vi "PianoPassiveBuzzer.vi"() -> ()   [LabVIEW 2024]
uses:
  Driver/CTIPicoVISA.lvlib
panel:
  in  "GroveConnector":enum16{"A0", "A1", "A2"}(ring)
  out "error out":errorcluster
  out "Identity":T1
  in  "Duty Cycle":dbl(slide)=0.09183673469387754 scale=0.0..1.0
  in  "D5#":bool
  in  "E5":bool
  in  "C5#":bool
  in  "D5":bool
  in  "A4#":bool
  in  "G4#":bool
  in  "F4#":bool
  in  "D4#":bool
  in  "C4#":bool
  in  "VISA resource":refnum<visa-resource-name>="ASRL5::INSTR"
  in  "stop":bool
  in  "C5":bool
  in  "B4":bool
  in  "A4":bool
  in  "G4":bool
  in  "F4":bool
  in  "E4":bool
  in  "D4":bool
  in  "C4":bool
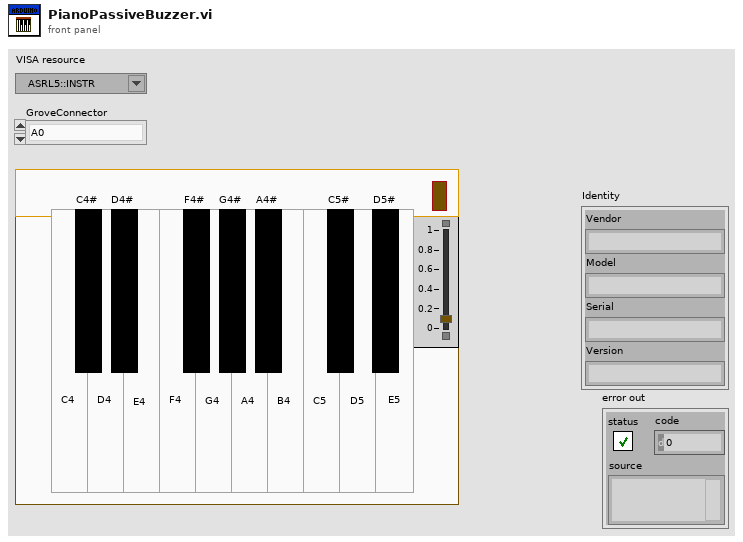
[diagram p1: front panel]
types:
  T1 = cluster{"Vendor":string, "Model":string, "Serial":string, "Version":string}
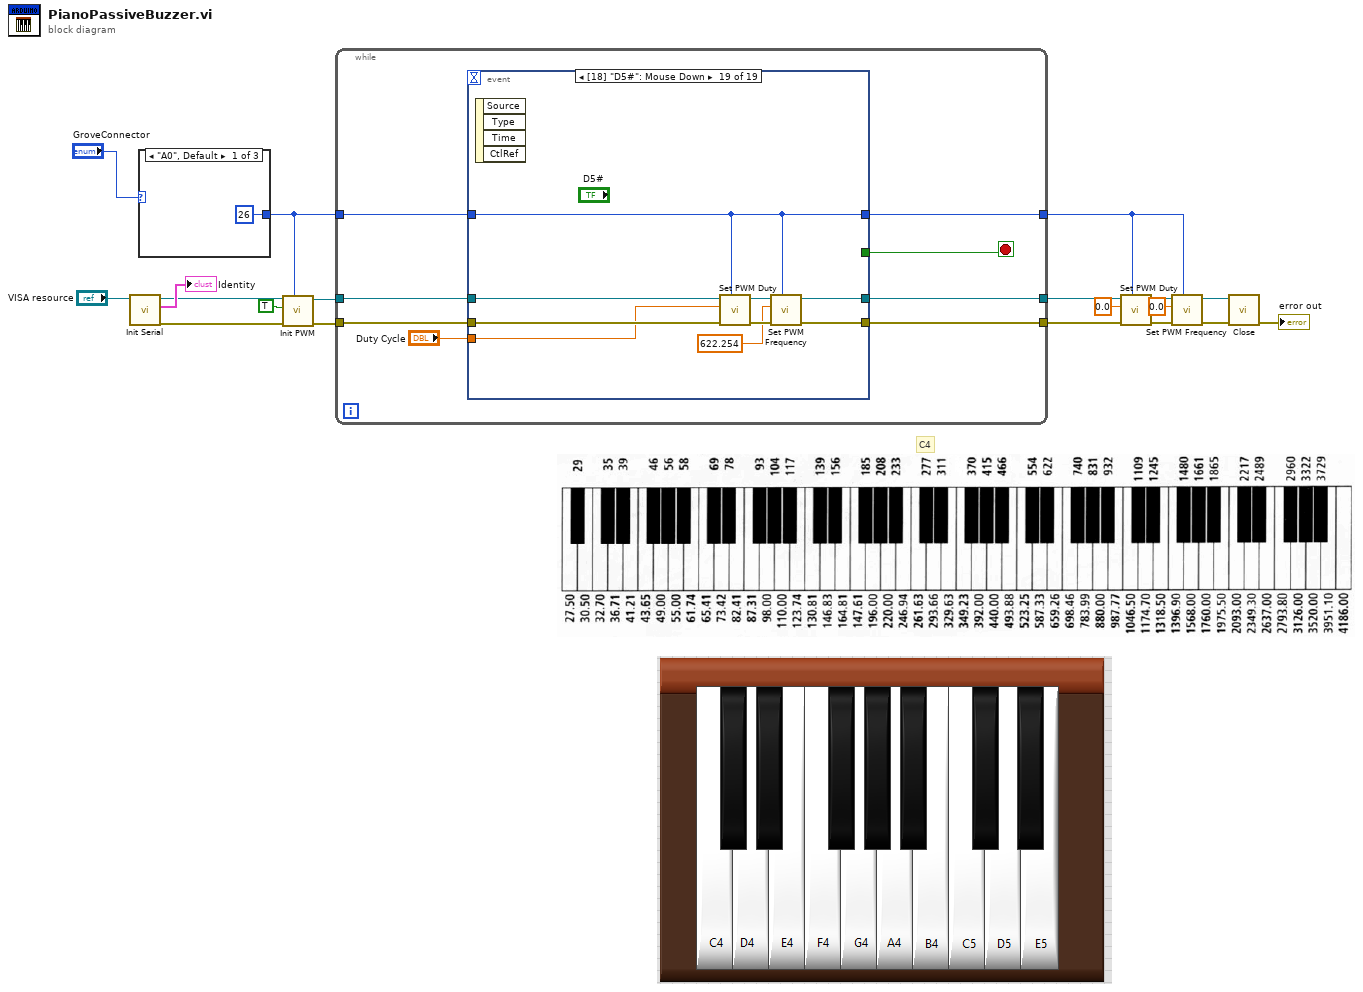
[diagram p0: block diagram]
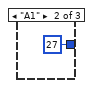
[diagram p2: hidden frame]
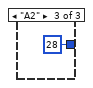
[diagram p3: hidden frame]
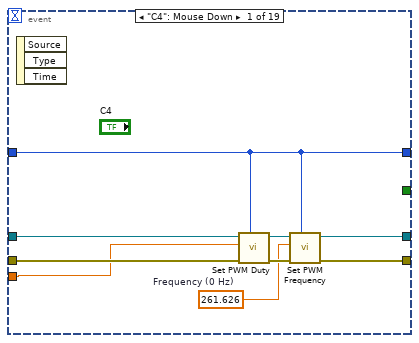
[diagram p4: hidden frame]
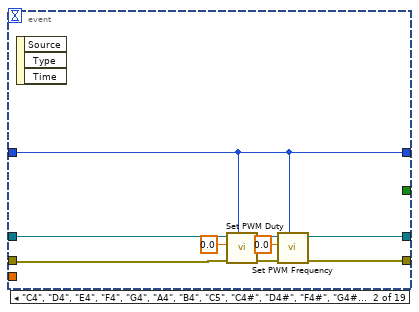
[diagram p5: hidden frame]
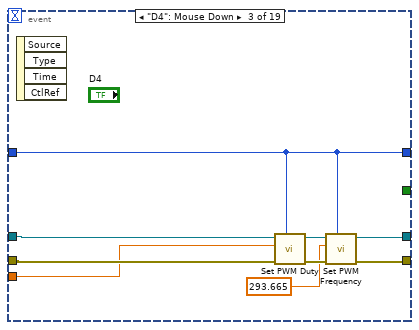
[diagram p6: hidden frame]
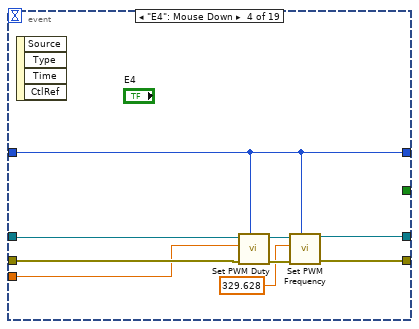
[diagram p7: hidden frame]
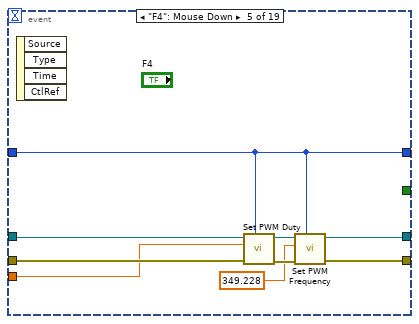
[diagram p8: hidden frame]
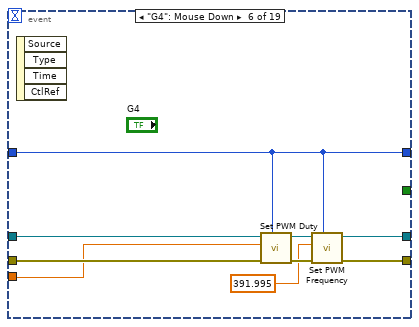
[diagram p9: hidden frame]
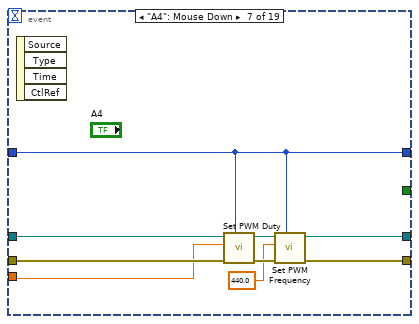
[diagram p10: hidden frame]
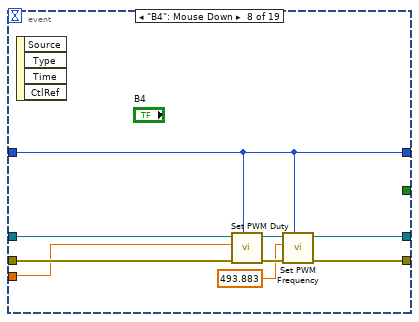
[diagram p11: hidden frame]
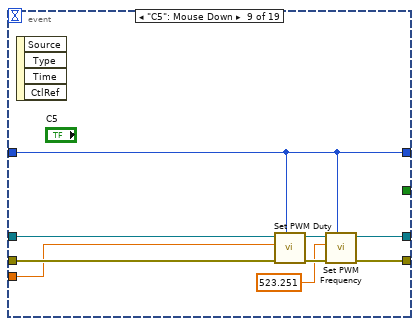
[diagram p12: hidden frame]
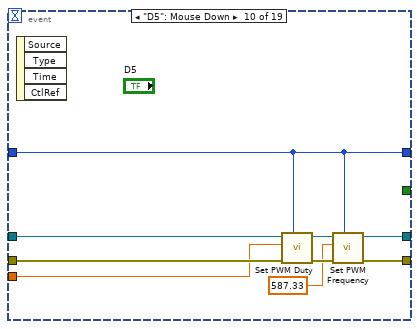
[diagram p13: hidden frame]
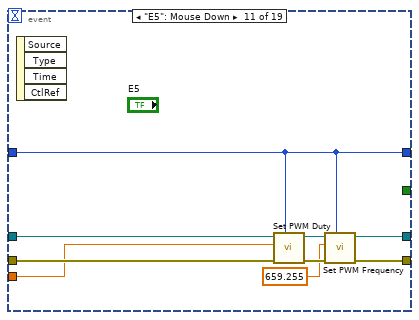
[diagram p14: hidden frame]
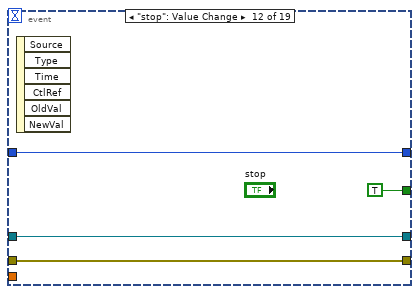
[diagram p15: hidden frame]
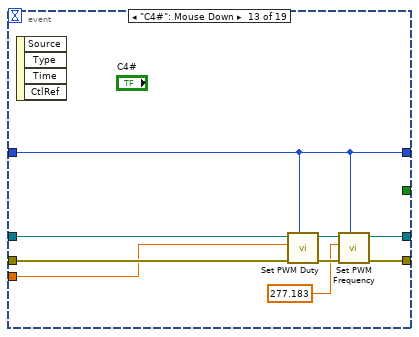
[diagram p16: hidden frame]
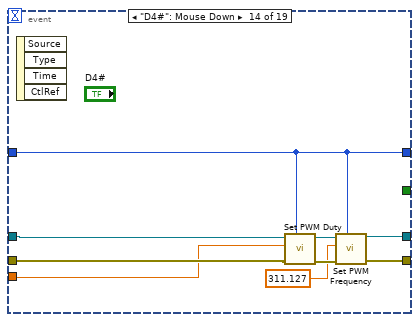
[diagram p17: hidden frame]
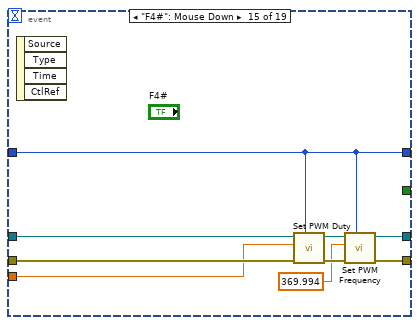
[diagram p18: hidden frame]
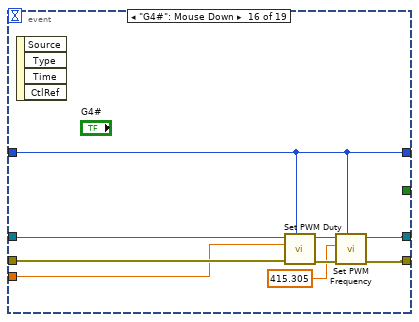
[diagram p19: hidden frame]
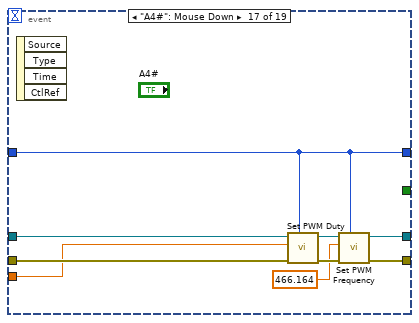
[diagram p20: hidden frame]
diagram:
  # "C4"
  n1 = call "Init Serial.vi"("VISA resource name in"="VISA resource") -> ("error out"=w12:errorcluster, "Identity"=→"Identity":T1, "VISA resource name Out"=w11:refnum<visa-resource-name>)  [unwired: 8 in]
  n2 = case shown="\"A0\", Default" "GroveConnector" {
    tunnel: [26 ("GPIO") 27 ("GPIO") 28 ("GPIO")] -> w2
    frame "A0", Default {
    }
    frame "A1" {
    }
    frame "A2" {
    }
  }
  n3 = call "Init PWM.vi"("GPIO"=w2, "error in (no error)"=w12, "Enable (F)"=TRUE, "VISA resource name in"=w11) -> ("error out"=w13:errorcluster, "VISA resource name"=w14:refnum<visa-resource-name>)  [unwired: 6 in]
  n4 = while {
    tunnel: w14 -> [w29]
    tunnel: w13 -> [w28]
    tunnel: [w25] -> w5
    tunnel: [w26] -> w6
    tunnel: w2 -> [w24]
    tunnel: [w23] -> w1
    stop <- w27 stop-if-true
    n5 = event shown="[18] \"D5#\": Mouse Down" {
      selector: _ -> [_ _ _ _ _ _ _ _ _ _ _ _ _ _ _ _ _ _ _]
      dyn-events: _ -> [_ _ _ _ _ _ _ _ _ _ _ _ _ _ _ _ _ _ _]
      timeout: _ -> [_ _ _ _ _ _ _ _ _ _ _ _ _ _ _ _ _ _ _]
      tunnel: "Duty Cycle" -> [w31 _ w49 w58 w68 w77 w85 w94 w103 w112 w122 _ w136 w144 w152 w162 w170 w179 w188]
      tunnel: w29 -> [w34 w44 w50 w62 w70 w79 w88 w98 w106 w115 w124 w132 w135 w146 w156 w164 w174 w183 w192]
      tunnel: w28 -> [w35 w43 w52 w61 w69 w78 w89 w97 w105 w114 w123 w131 w137 w145 w155 w163 w173 w182 w191]
      tunnel: [w36 w45 w54 w63 w72 w81 w90 w99 w108 w116 w126 w131 w139 w148 w157 w166 w175 w184 w193] -> w25
      tunnel: [w37 w46 w55 w64 w73 w82 w91 w100 w109 w118 w127 w132 w140 w149 w158 w167 w176 w185 w194] -> w26
      tunnel: [_ _ _ _ _ _ _ _ _ _ _ TRUE _ _ _ _ _ _ _] -> w27
      tunnel: w24 -> [w33 w40 w53 w60 w71 w80 w87 w96 w107 w117 w125 w130 w134 w147 w154 w165 w172 w181 w190]
      tunnel: [w33 w40 w53 w60 w71 w80 w87 w96 w107 w117 w125 w130 w134 w147 w154 w165 w172 w181 w190] -> w23
      event "C4": Mouse Down {
        w32 = 261.626  # Frequency (0 Hz)
        n6 = event-data() -> ()  [unwired: 1 in, 3 out]
        n7 = call "Set PWM Duty.vi"("GPIO"=w33, "error in (no error)"=w35, "Duty % (0-1)"=w31, "VISA resource name in"=w34) -> ("error out"=w39:errorcluster, "VISA resource name"=w38:refnum<visa-resource-name>)  [unwired: 6 in]
        n8 = call "Set PWM Frequency.vi"("GPIO"=w33, "error in (no error)"=w39, "Freq Hz"=w32, "VISA resource name in"=w38) -> ("error out"=w36:errorcluster, "VISA resource name"=w37:refnum<visa-resource-name>)  [unwired: 6 in]
      }
      event "C4", "D4", "E4", "F4", "G4", "A4", "B4", "C5", "C4#", "D4#", "F4#", "G4#", "A4#", "C5#", "D5", "D5#", "E5": Mouse Up {
        n9 = event-data() -> ()  [unwired: 1 in, 3 out]
        n10 = call "Set PWM Duty.vi"("GPIO"=w40, "error in (no error)"=w43, "Duty % (0-1)"=sgl 0.0, "VISA resource name in"=w44) -> ("error out"=w48:errorcluster, "VISA resource name"=w47:refnum<visa-resource-name>)  [unwired: 6 in]
        n11 = call "Set PWM Frequency.vi"("GPIO"=w40, "error in (no error)"=w48, "Freq Hz"=sgl 0.0, "VISA resource name in"=w47) -> ("error out"=w45:errorcluster, "VISA resource name"=w46:refnum<visa-resource-name>)  [unwired: 6 in]
      }
      event "D4": Mouse Down {
        n12 = event-data() -> ()  [unwired: 1 in, 4 out]
        n13 = call "Set PWM Duty.vi"("GPIO"=w53, "error in (no error)"=w52, "Duty % (0-1)"=w49, "VISA resource name in"=w50) -> ("error out"=w57:errorcluster, "VISA resource name"=w56:refnum<visa-resource-name>)  [unwired: 6 in]
        n14 = call "Set PWM Frequency.vi"("GPIO"=w53, "error in (no error)"=w57, "Freq Hz"=293.665 ("Frequency (0 Hz)"), "VISA resource name in"=w56) -> ("error out"=w54:errorcluster, "VISA resource name"=w55:refnum<visa-resource-name>)  [unwired: 6 in]
      }
      event "E4": Mouse Down {
        n15 = event-data() -> ()  [unwired: 1 in, 4 out]
        n16 = call "Set PWM Duty.vi"("GPIO"=w60, "error in (no error)"=w61, "Duty % (0-1)"=w58, "VISA resource name in"=w62) -> ("error out"=w66:errorcluster, "VISA resource name"=w65:refnum<visa-resource-name>)  [unwired: 6 in]
        n17 = call "Set PWM Frequency.vi"("GPIO"=w60, "error in (no error)"=w66, "Freq Hz"=329.628 ("Frequency (0 Hz)"), "VISA resource name in"=w65) -> ("error out"=w63:errorcluster, "VISA resource name"=w64:refnum<visa-resource-name>)  [unwired: 6 in]
      }
      event "F4": Mouse Down {
        n18 = event-data() -> ()  [unwired: 1 in, 4 out]
        n19 = call "Set PWM Duty.vi"("GPIO"=w71, "error in (no error)"=w69, "Duty % (0-1)"=w68, "VISA resource name in"=w70) -> ("error out"=w75:errorcluster, "VISA resource name"=w74:refnum<visa-resource-name>)  [unwired: 6 in]
        n20 = call "Set PWM Frequency.vi"("GPIO"=w71, "error in (no error)"=w75, "Freq Hz"=349.228, "VISA resource name in"=w74) -> ("error out"=w72:errorcluster, "VISA resource name"=w73:refnum<visa-resource-name>)  [unwired: 6 in]
      }
      event "G4": Mouse Down {
        n21 = event-data() -> ()  [unwired: 1 in, 4 out]
        n22 = call "Set PWM Duty.vi"("GPIO"=w80, "error in (no error)"=w78, "Duty % (0-1)"=w77, "VISA resource name in"=w79) -> ("error out"=w84:errorcluster, "VISA resource name"=w83:refnum<visa-resource-name>)  [unwired: 6 in]
        n23 = call "Set PWM Frequency.vi"("GPIO"=w80, "error in (no error)"=w84, "Freq Hz"=391.995, "VISA resource name in"=w83) -> ("error out"=w81:errorcluster, "VISA resource name"=w82:refnum<visa-resource-name>)  [unwired: 6 in]
      }
      event "A4": Mouse Down {
        n24 = event-data() -> ()  [unwired: 1 in, 4 out]
        n25 = call "Set PWM Duty.vi"("GPIO"=w87, "error in (no error)"=w89, "Duty % (0-1)"=w85, "VISA resource name in"=w88) -> ("error out"=w93:errorcluster, "VISA resource name"=w92:refnum<visa-resource-name>)  [unwired: 6 in]
        n26 = call "Set PWM Frequency.vi"("GPIO"=w87, "error in (no error)"=w93, "Freq Hz"=440.0, "VISA resource name in"=w92) -> ("error out"=w90:errorcluster, "VISA resource name"=w91:refnum<visa-resource-name>)  [unwired: 6 in]
      }
      event "B4": Mouse Down {
        n27 = event-data() -> ()  [unwired: 1 in, 4 out]
        n28 = call "Set PWM Duty.vi"("GPIO"=w96, "error in (no error)"=w97, "Duty % (0-1)"=w94, "VISA resource name in"=w98) -> ("error out"=w102:errorcluster, "VISA resource name"=w101:refnum<visa-resource-name>)  [unwired: 6 in]
        n29 = call "Set PWM Frequency.vi"("GPIO"=w96, "error in (no error)"=w102, "Freq Hz"=493.883, "VISA resource name in"=w101) -> ("error out"=w99:errorcluster, "VISA resource name"=w100:refnum<visa-resource-name>)  [unwired: 6 in]
      }
      event "C5": Mouse Down {
        n30 = event-data() -> ()  [unwired: 1 in, 4 out]
        n31 = call "Set PWM Duty.vi"("GPIO"=w107, "error in (no error)"=w105, "Duty % (0-1)"=w103, "VISA resource name in"=w106) -> ("error out"=w111:errorcluster, "VISA resource name"=w110:refnum<visa-resource-name>)  [unwired: 6 in]
        n32 = call "Set PWM Frequency.vi"("GPIO"=w107, "error in (no error)"=w111, "Freq Hz"=523.251, "VISA resource name in"=w110) -> ("error out"=w108:errorcluster, "VISA resource name"=w109:refnum<visa-resource-name>)  [unwired: 6 in]
      }
      event "D5": Mouse Down {
        n33 = event-data() -> ()  [unwired: 1 in, 4 out]
        n34 = call "Set PWM Duty.vi"("GPIO"=w117, "error in (no error)"=w114, "Duty % (0-1)"=w112, "VISA resource name in"=w115) -> ("error out"=w120:errorcluster, "VISA resource name"=w119:refnum<visa-resource-name>)  [unwired: 6 in]
        n35 = call "Set PWM Frequency.vi"("GPIO"=w117, "error in (no error)"=w120, "Freq Hz"=587.33, "VISA resource name in"=w119) -> ("error out"=w116:errorcluster, "VISA resource name"=w118:refnum<visa-resource-name>)  [unwired: 6 in]
      }
      event "E5": Mouse Down {
        n36 = event-data() -> ()  [unwired: 1 in, 4 out]
        n37 = call "Set PWM Duty.vi"("GPIO"=w125, "error in (no error)"=w123, "Duty % (0-1)"=w122, "VISA resource name in"=w124) -> ("error out"=w129:errorcluster, "VISA resource name"=w128:refnum<visa-resource-name>)  [unwired: 6 in]
        n38 = call "Set PWM Frequency.vi"("GPIO"=w125, "error in (no error)"=w129, "Freq Hz"=659.255, "VISA resource name in"=w128) -> ("error out"=w126:errorcluster, "VISA resource name"=w127:refnum<visa-resource-name>)  [unwired: 6 in]
      }
      event "stop": Value Change {
        n39 = event-data() -> ()  [unwired: 1 in, 6 out]
      }
      event "C4#": Mouse Down {
        n40 = event-data() -> ()  [unwired: 1 in, 4 out]
        n41 = call "Set PWM Duty.vi"("GPIO"=w134, "error in (no error)"=w137, "Duty % (0-1)"=w136, "VISA resource name in"=w135) -> ("error out"=w142:errorcluster, "VISA resource name"=w141:refnum<visa-resource-name>)  [unwired: 6 in]
        n42 = call "Set PWM Frequency.vi"("GPIO"=w134, "error in (no error)"=w142, "Freq Hz"=277.183, "VISA resource name in"=w141) -> ("error out"=w139:errorcluster, "VISA resource name"=w140:refnum<visa-resource-name>)  [unwired: 6 in]
      }
      event "D4#": Mouse Down {
        n43 = event-data() -> ()  [unwired: 1 in, 4 out]
        n44 = call "Set PWM Duty.vi"("GPIO"=w147, "error in (no error)"=w145, "Duty % (0-1)"=w144, "VISA resource name in"=w146) -> ("error out"=w151:errorcluster, "VISA resource name"=w150:refnum<visa-resource-name>)  [unwired: 6 in]
        n45 = call "Set PWM Frequency.vi"("GPIO"=w147, "error in (no error)"=w151, "Freq Hz"=311.127, "VISA resource name in"=w150) -> ("error out"=w148:errorcluster, "VISA resource name"=w149:refnum<visa-resource-name>)  [unwired: 6 in]
      }
      event "F4#": Mouse Down {
        n46 = event-data() -> ()  [unwired: 1 in, 4 out]
        n47 = call "Set PWM Duty.vi"("GPIO"=w154, "error in (no error)"=w155, "Duty % (0-1)"=w152, "VISA resource name in"=w156) -> ("error out"=w160:errorcluster, "VISA resource name"=w159:refnum<visa-resource-name>)  [unwired: 6 in]
        n48 = call "Set PWM Frequency.vi"("GPIO"=w154, "error in (no error)"=w160, "Freq Hz"=369.994, "VISA resource name in"=w159) -> ("error out"=w157:errorcluster, "VISA resource name"=w158:refnum<visa-resource-name>)  [unwired: 6 in]
      }
      event "G4#": Mouse Down {
        n49 = event-data() -> ()  [unwired: 1 in, 4 out]
        n50 = call "Set PWM Duty.vi"("GPIO"=w165, "error in (no error)"=w163, "Duty % (0-1)"=w162, "VISA resource name in"=w164) -> ("error out"=w169:errorcluster, "VISA resource name"=w168:refnum<visa-resource-name>)  [unwired: 6 in]
        n51 = call "Set PWM Frequency.vi"("GPIO"=w165, "error in (no error)"=w169, "Freq Hz"=415.305, "VISA resource name in"=w168) -> ("error out"=w166:errorcluster, "VISA resource name"=w167:refnum<visa-resource-name>)  [unwired: 6 in]
      }
      event "A4#": Mouse Down {
        n52 = event-data() -> ()  [unwired: 1 in, 4 out]
        n53 = call "Set PWM Duty.vi"("GPIO"=w172, "error in (no error)"=w173, "Duty % (0-1)"=w170, "VISA resource name in"=w174) -> ("error out"=w178:errorcluster, "VISA resource name"=w177:refnum<visa-resource-name>)  [unwired: 6 in]
        n54 = call "Set PWM Frequency.vi"("GPIO"=w172, "error in (no error)"=w178, "Freq Hz"=466.164, "VISA resource name in"=w177) -> ("error out"=w175:errorcluster, "VISA resource name"=w176:refnum<visa-resource-name>)  [unwired: 6 in]
      }
      event "C5#": Mouse Down {
        n55 = event-data() -> ()  [unwired: 1 in, 4 out]
        n56 = call "Set PWM Duty.vi"("GPIO"=w181, "error in (no error)"=w182, "Duty % (0-1)"=w179, "VISA resource name in"=w183) -> ("error out"=w187:errorcluster, "VISA resource name"=w186:refnum<visa-resource-name>)  [unwired: 6 in]
        n57 = call "Set PWM Frequency.vi"("GPIO"=w181, "error in (no error)"=w187, "Freq Hz"=554.365, "VISA resource name in"=w186) -> ("error out"=w184:errorcluster, "VISA resource name"=w185:refnum<visa-resource-name>)  [unwired: 6 in]
      }
      event "D5#": Mouse Down {
        n58 = event-data() -> ()  [unwired: 1 in, 4 out]
        n59 = call "Set PWM Duty.vi"("GPIO"=w190, "error in (no error)"=w191, "Duty % (0-1)"=w188, "VISA resource name in"=w192) -> ("error out"=w196:errorcluster, "VISA resource name"=w195:refnum<visa-resource-name>)  [unwired: 6 in]
        n60 = call "Set PWM Frequency.vi"("GPIO"=w190, "error in (no error)"=w196, "Freq Hz"=622.254, "VISA resource name in"=w195) -> ("error out"=w193:errorcluster, "VISA resource name"=w194:refnum<visa-resource-name>)  [unwired: 6 in]
      }
    }
  }
  n61 = call "Set PWM Duty.vi"("GPIO"=w1, "error in (no error)"=w5, "Duty % (0-1)"=sgl 0.0, "VISA resource name in"=w6) -> ("error out"=w7:errorcluster, "VISA resource name"=w8:refnum<visa-resource-name>)  [unwired: 6 in]
  n62 = call "Set PWM Frequency.vi"("GPIO"=w1, "error in (no error)"=w7, "Freq Hz"=sgl 0.0, "VISA resource name in"=w8) -> ("error out"=w3:errorcluster, "VISA resource name"=w4:refnum<visa-resource-name>)  [unwired: 6 in]
  n63 = call "Close.vi"("error in (no error)"=w3, "VISA resource name in"=w4) -> ("error out"=→"error out":errorcluster)  [unwired: 9 in]
